vi "Overlay.vi"(8 "error in (no error)":errorcluster, 10 "Image In":T1, 11 "Overlay Base in":refnum<class "Analyze Results q-Factor.lvclass">) -> (0 "error out":errorcluster, 2 "Image out":T1, 3 "Overlay Base out":refnum<class "Analyze Results q-Factor.lvclass">)   [LabVIEW 2014, in "Analyze Results q-Factor.lvclass"]
uses:
  Analyze Results q-Factor.lvclass
  <vilib>/vision/Image Controls.llb/IMAQ Image.ctl
  Results Base/Analyze Results Base.lvclass/Analyze Results Base.ctl
  Analyze Results q-Factor.lvclass/Analyze Results q-Factor.ctl
  Results Base/Read Overlay_.vi
  Read Focus ROI.vi
  Read q.vi
  Read Width Method.vi
  Read A.vi
  Results Base/Read Overlay colors.vi
  Results Base/Read Font, Size & Style.vi
  Results Base/Analyze Results Base.lvclass
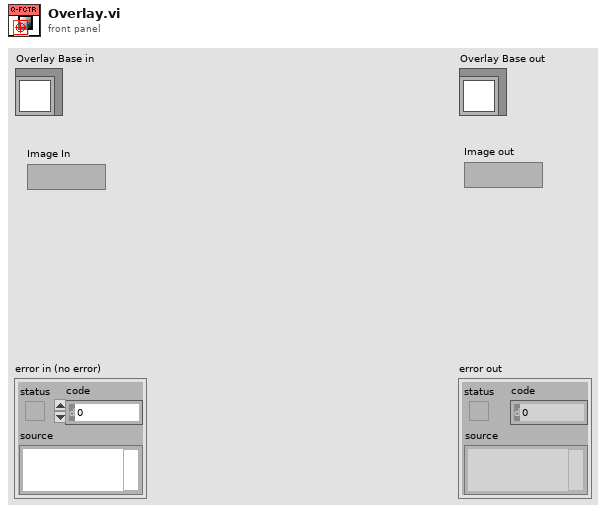
[diagram p1: front panel]
types:
  T1 = typedef "IMAQ Image.ctl" = refnum<image>
  T2 = typedef "ROI Descriptor" = cluster{"Global Rectangle":i32[], "Contours":cluster{"ID":enum32{"External", "Internal"}, "Type":u32, "Coordinates":i32[]}[]}
  T3 = cluster{"Desired Font (Application)":enum16{"User-specified Font", "Application Font", "System Font", "Dialog Font"}, "[User-specified Font]":cluster{"Font Name":string, "Size":i16, "Strikeout?":bool, "Italic?":bool, "Underline?":bool, "Outline?":bool, "Shadow?":bool, "Bold?":bool, "Rotation Angle":dbl}, "Horizontal Alignment":i16, "Vertical Alignment":i16}
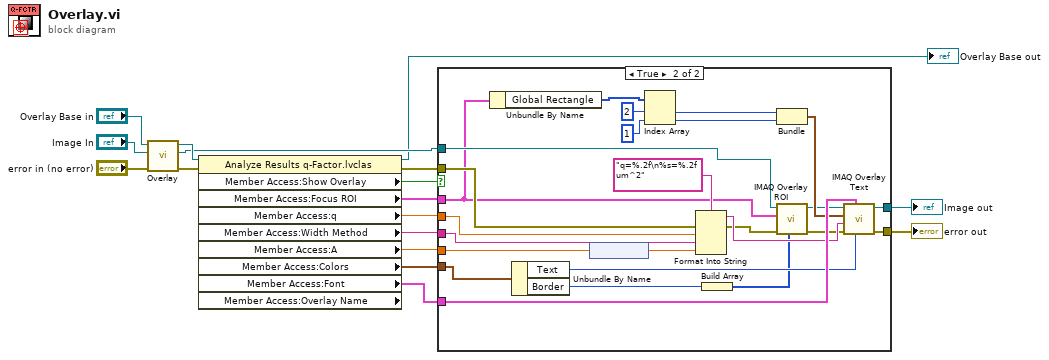
[diagram p0: block diagram]
diagram:
  n1 = call-parent "Overlay.vi"("error in (no error)"="error in (no error)", "Image In"="Image In", "Overlay Base in"="Overlay Base in") -> ("error out"=w12:errorcluster, "Image out"=w8:T1, "Overlay Base out"=w14:refnum<class "Analyze Results q-Factor.lvclass">)  [unwired: 6 in]
  n2 = property class="Analyze Results q-Factor.lvclas" props=["Member Access:Show Overlay", "Member Access:Focus ROI", "Member Access:q", "Member Access:Width Method", "Member Access:A", "Member Access:Colors", "Member Access:Font", "Member Access:Overlay Name"](reference=w14, error in=w12) -> (reference out=→"Overlay Base out":refnum<class "Analyze Results q-Factor.lvclass">, error out=w11:errorcluster, "Member Access:Show Overlay"=w13:bool, "Member Access:Focus ROI"=w7:T2, "Member Access:q"=w6:dbl, "Member Access:Width Method"=w5:string, "Member Access:A"=w4:dbl[unit], "Member Access:Colors"=w1:cluster{"Border":u32, "Text":u32}, "Member Access:Font"=w2:T3)  [unwired: 1 out]
  n3 = case shown="True" w13 {
    tunnel: w8 -> [w19 w38]
    tunnel: [w19 w42] -> w9
    tunnel: w11 -> [w18 w24]
    tunnel: [w18 w41] -> w10
    tunnel: w7 -> [_ w22]
    tunnel: w6 -> [_ w27]
    tunnel: w5 -> [_ w26]
    tunnel: w4 -> [_ w25]
    tunnel: w2 -> [_ w44]
    tunnel: w1 -> [_ w21]
    frame False {
    }
    frame True {
      n4 = Unbundle By Name(w22) -> ("Global Rectangle"=w32:i32[])
      n5 = Unbundle By Name(w21) -> ("Text"=w40:u32, "Border"=w36:u32)
      n6 = node(w25) -> (w20:dbl)
      n7 = Index Array(array=w32, index #1=2 ("index"), index #2=1 ("index")) -> (element #1=w34:i32, element #2=w33:i32)
      n8 = Format Into String(format string="q=%.2f\n%s=%.2f um^2", error in=w24, w27, w26, w20) -> (resulting string=w43:string, error out=w23:errorcluster)  [unwired: 1 in]
      n9 = Build Array(w36) -> (w35:u32[])
      n10 = Bundle(w34, w33) -> (w39:cluster{i32, i32})  [unwired: 1 in]
      n11 = call "IMAQ Overlay ROI"("Colors (Green)"=w35, "error in (no error)"=w23, "ROI Descriptor"=w22, "Image"=w38) -> ("error out"=w29:errorcluster, "Image Out"=w37:T1)  [unwired: 6 in]
      n12 = call "IMAQ Overlay Text"("Text Color (black)"=w40, "Font, Size & Style"=w44, "error in (no error)"=w29, "String"=w43, "Origin"=w39, "Image"=w37) -> ("error out"=w41:errorcluster, "Image Out"=w42:T1)  [unwired: 4 in]
    }
  }
  "error out" <- w10
  "Image out" <- w9
